vi "角度至弧度1D（单位）.vi"(1 "degrees":dbl[unit][](array[numeric]) format="%.2f") -> (0 "radians":dbl[unit][](array[numeric]) format="%.2f")   [LabVIEW 2012, in "几何工具.lvlib"]
doc: "功能：\n\n一维数组角度转换为弧度。\n\n输入：角度，单位为度。\n\n输出：弧度。\n\ncsxcs_366创建。"
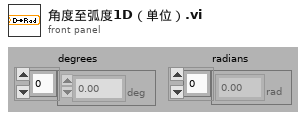
[diagram p1: front panel]
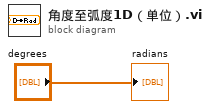
[diagram p0: block diagram]
diagram:
  "radians" <- "degrees"
